vi "Actor Core.vi"(8 "error in":errorcluster, 11 "Nested in":refnum<class "Interactor.lvclass">) -> (0 "error out":errorcluster, 3 "Actor out":refnum<class "Actor.lvclass">)   [LabVIEW 2024, in "Interactor.lvlib" / "Interactor.lvclass"]
doc: "(<B>Filename</B>: Actor Framework.lvlib:Actor.lvclass:Actor Core.vi)\n\nReceives messages to the actor, reacts to them, and initiates any error handling that may shut the actor down.\n\nDescendant classes may override this VI to append parallel tasks for the actor to complete while it handles messages. Overrides use the Call Parent Method node."
uses:
  Interactor.lvclass
  <vilib>/ActorFramework/Actor/Actor.lvclass
  Object Dictionary UI/Object Dictionary UI.lvclass
  Home/Home.lvclass
  Interactor.lvclass/Interactor.ctl
  <vilib>/MGI/Panel Manager/Panel/Panel/Subpanel/Subpanel.lvclass
  <vilib>/ActorFramework/Stop Msg/Stop Msg.lvclass
  Interactor Messages/Show Nested Panel Msg/Show Nested Panel Msg.lvclass
  Interactor Messages/Publish Discovered Nodes Msg/Publish Discovered Nodes Msg.lvclass
  <vilib>/MGI/Panel Manager/Panel Actor/Panel Actor/Panel Actor.lvclass
  <vilib>/MGI/Panel Manager/Panel/Panel.lvlib
  CANopen Master/CANopen Master.lvclass
  HAL/Source/Instrument Manager/Instrument Manager.lvclass
  <vilib>/MGI/Panel Manager/Panel/Panel/Subpanel/Subpanel.vi
panel:
  in  "Copy Log Button":bool
  out "Communication Log":string
  in  "Object Dictionary":bool
  in  "Home Button":bool
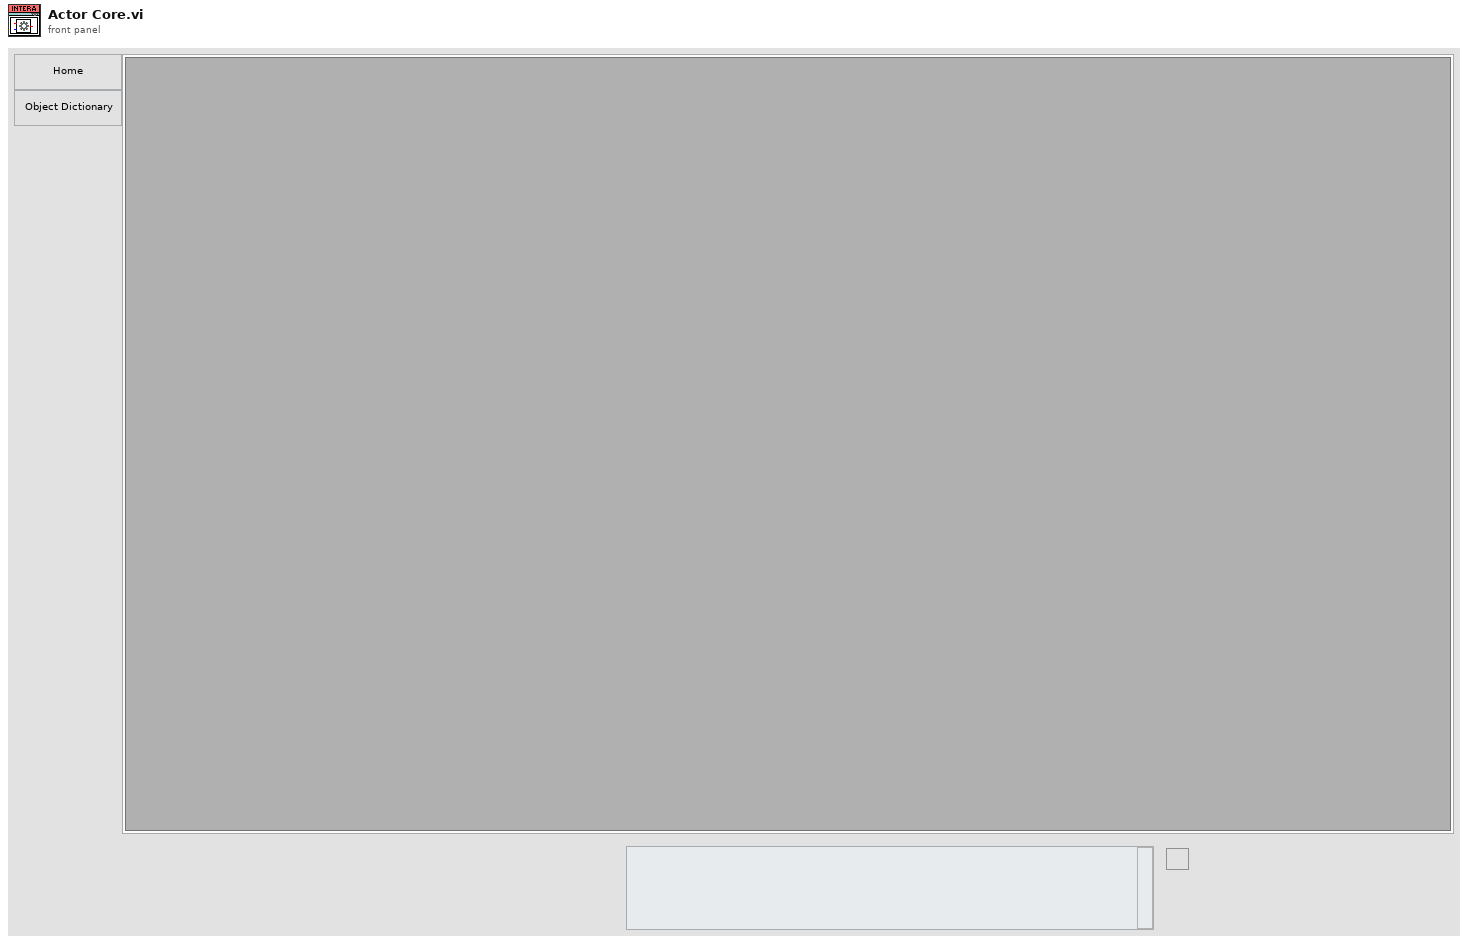
[diagram p1: front panel]
types:
  T1 = cluster{"Stop":refnum<user-event>, "Msg Sent Source":refnum<user-event>}
  T2 = cluster{"Stop CAN Task":refnum<user-event>, "Msg Received":refnum<user-event>, "CAN Task Error":refnum<user-event>, "Node Discovered":refnum<user-event>}
  T3 = cluster{"Pnl Actor":refnum<event-registration>, "Event Registration Refnum":refnum<event-registration>}
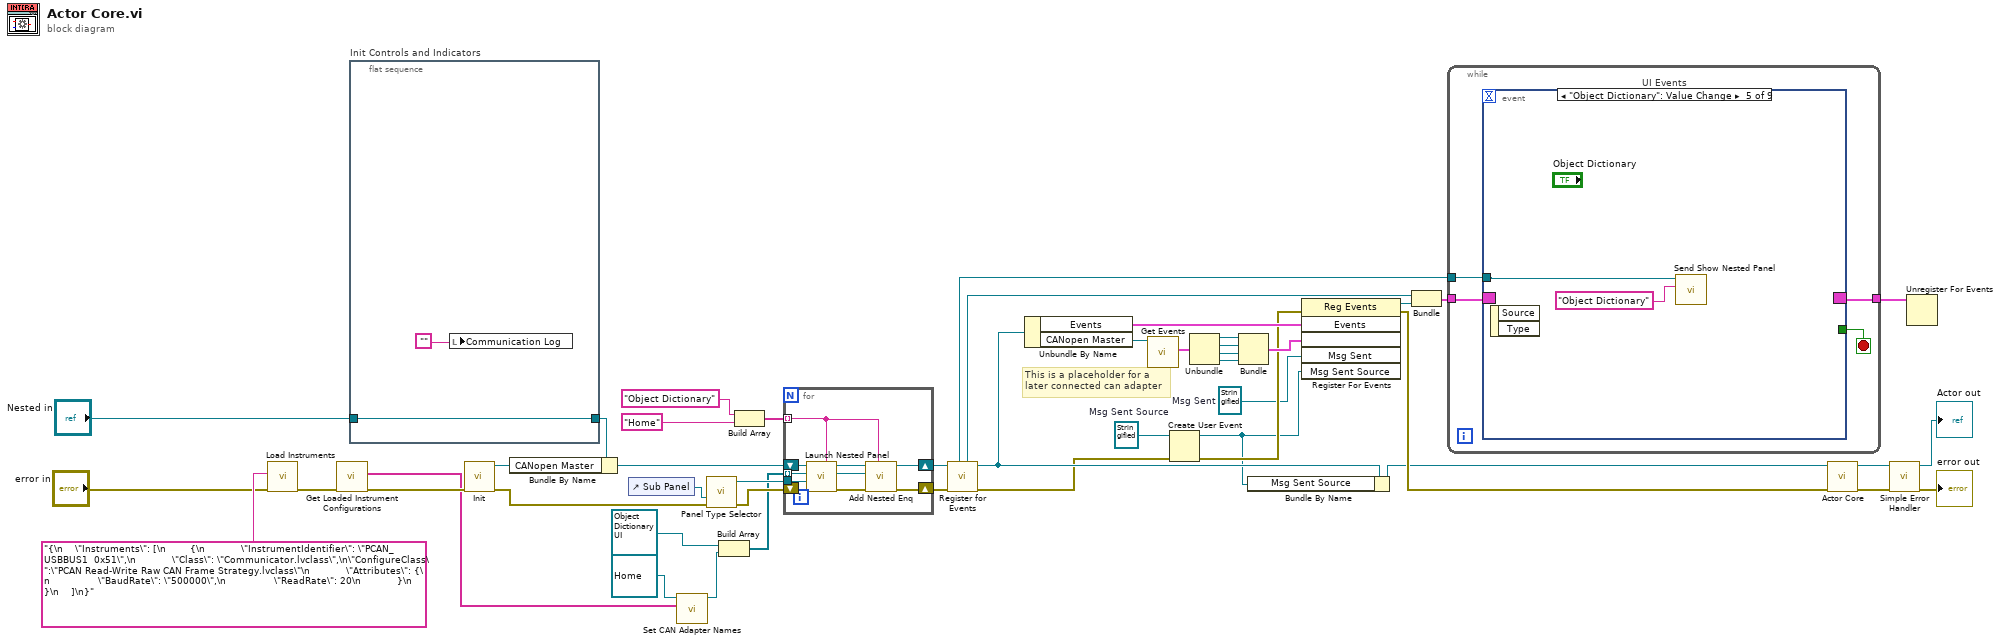
[diagram p0: block diagram]
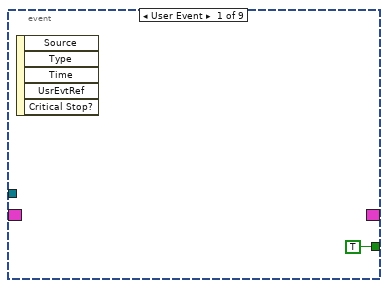
[diagram p2: hidden frame]
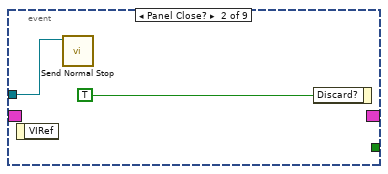
[diagram p3: hidden frame]
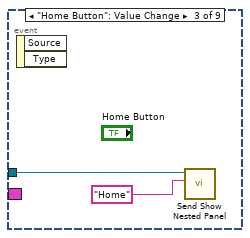
[diagram p4: hidden frame]
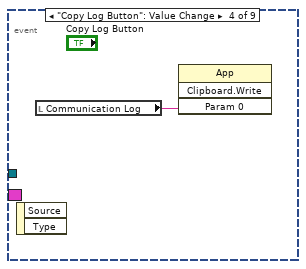
[diagram p5: hidden frame]
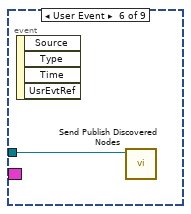
[diagram p6: hidden frame]
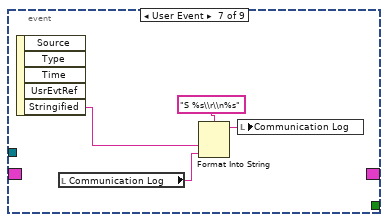
[diagram p7: hidden frame]
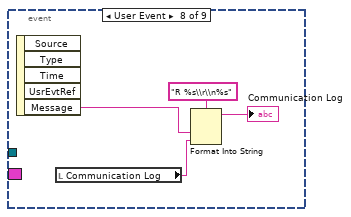
[diagram p8: hidden frame]
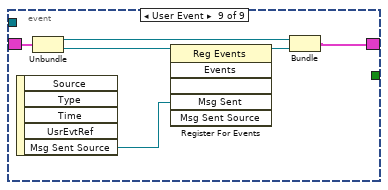
[diagram p9: hidden frame]
diagram:
  w5 = refnum<user-event> refnum  # Msg Sent Source
  w6 = refnum<user-event> refnum  # Msg Sent
  # "This is a placeholder for a\nlater connected can adapter"
  n1 = call "Load Instruments.vi"("Error In"="error in", "Source"="{\n    \"Instruments\": [\n        {\n            \"InstrumentIdentifier\": \"PCAN_USBBUS1  0x51\",\n            \"Class\": \"Communicator.lvclass\",\n\"ConfigureClass\":\"PCAN Read-Write Raw CAN Frame Strategy.lvclass\"\n            \"Attributes\": {\n                \"BaudRate\": \"500000\",\n                \"ReadRate\": 20\n            }\n        }\n    ]\n}" ("<JSON>CFG")) -> ("Error Out"=w13:errorcluster)  [unwired: 9 in]
  n2 = call "Get Loaded Instrument Configurations.vi"("Error In"=w13) -> ("Error Out"=w17:errorcluster, "Identifiers"=w16:string[])  [unwired: 8 in, 1 out]
  n3 = flat-sequence "Init Controls and Indicators" {
    tunnel: "Nested in" -> [w48]
    tunnel: [w48] -> w22
    frame #0 {
      n4 = local write "Communication Log"("") -> ()
    }
  }
  n5 = call "Init.vi"("error in"=w17) -> ("error out"=w19:errorcluster, "CANopen Master out"=w21:refnum<class "CANopen Master.lvclass">)  [unwired: 9 in]
  n6 = Bundle By Name(cluster=w22, "CANopen Master"=w21) -> (w20:refnum<class "Interactor.lvclass">)
  n7 = control-ref of="Sub Panel"() -> (w39:refnum<vi>)
  n8 = call "Set CAN Adapter Names.vi"("ICommunicate Names"=w16, "Home in"=refnum<class "Home.lvclass"> refnum) -> ("Home out"=w28:refnum<class "Home.lvclass">)  [unwired: 9 in]
  n9 = call-poly <vilib>:"Panel Type Selector.vi"("Error In"=w19, "Sub Panel"=w39) -> ("Error Out"=w38:errorcluster, "Subpanel Out"=w34:refnum<class "Subpanel.lvclass">)  [unwired: 8 in]
  n10 = Build Array(refnum<class "Object Dictionary UI.lvclass"> refnum ("Object Dictionary.lvlib:Object Dictionary.lvclass"), w28) -> (w33:refnum<class "Panel Actor.lvclass">[])
  n11 = Build Array("Object Dictionary" ("Debug Alias"), "Home" ("Debug Alias")) -> (w32:string[])
  n12 = for {
    tunnel: w34 -> [w51]
    shift-right: [w55] -> w37
    shift-left: w38 -> [w57]
    shift-right: [w52] -> w35
    shift-left: w20 -> [w56]
    tunnel: w33 -> [w50] mode=indexing
    tunnel: w32 -> [w49] mode=indexing
    n13 = call <vilib>:"Launch Nested Panel.vi"("Debug Alias"=w49, "error in (no error)"=w57, "Panel"=w51, "Nested Panel Actor"=w50, "Panel Actor in"=w56) -> ("error out"=w55:errorcluster, "Nested Actor's Enqueuer"=w53:refnum<class "Message Enqueuer.lvclass">, "Panel Actor out"=w54:refnum<class "Interactor.lvclass">)  [unwired: 3 in, 1 out]
    n14 = call "Add Nested Enq.vi"("Ident"=w49, "Nested Actor's Enqueuer"=w53, "Interactor in"=w54) -> ("Interactor out"=w52:refnum<class "Interactor.lvclass">)  [unwired: 8 in]
  }
  n15 = call <vilib>:"Register for Events.vi"("Error In"=w37, "Panel Actor in"=w35) -> ("Error Out"=w8:errorcluster, "Panel Actor out"=w36:refnum<class "Interactor.lvclass">, "Pnl Actor"=w40:refnum<event-registration>, "Self Enqueuer"=w43:refnum<class "Message Enqueuer.lvclass">)  [unwired: 6 in]
  n16 = Unbundle By Name(w36) -> ("Events"=w27:T1, "CANopen Master"=w23:refnum<class "CANopen Master.lvclass">)
  n17 = call "Get Events.vi"("CANopen Master in"=w23) -> ("Events"=w25:T2)  [unwired: 9 in, 1 out]
  n18 = Create User Event(user event datatype=w5, error in=w8) -> (user event=w3:refnum<user-event>, error out=w7:errorcluster)
  n19 = Unbundle(w25) -> ("Stop CAN Task"=w12:refnum<user-event>, "Msg Received"=w11:refnum<user-event>, "CAN Task Error"=w10:refnum<user-event>, "Node Discovered"=w9:refnum<user-event>)
  n20 = Bundle("Stop CAN Task"=w12, "Msg Received"=w11, "CAN Task Error"=w10, "Node Discovered"=w9) -> (w24:T2)  [unwired: 1 in]
  n21 = Bundle By Name(cluster=w36, "Msg Sent Source"=w3) -> (w4:refnum<class "Interactor.lvclass">)
  n22 = register-events ("Main Register for Events")(error in=w7, w27, w24, w6, w3) -> (reference out=w41:refnum<event-registration>, error out=w26:errorcluster)  [unwired: 1 in]
  n23 = Bundle("Pnl Actor"=w40, "Event Registration Refnum"=w41) -> (w42:T3)  [unwired: 1 in]
  n24 = while {
    tunnel: w42 -> [w61]
    tunnel: [w59] -> w44
    tunnel: w43 -> [w58]
    stop <- w60 stop-if-true
    n25 = event "UI Events" shown="[4] \"Object Dictionary\": Value Change" {
      selector: w61 -> [_ _ _ _ _ _ _ _ w84]
      dyn-events: [_ _ _ _ _ _ _ _ w79] -> w59
      timeout: _ -> [_ _ _ _ _ _ _ _ _]
      tunnel: [TRUE _ _ _ _ _ _ _ _] -> w60
      tunnel: w58 -> [_ w63 w66 _ w68 w70 _ _ _]
      event User Event {
        n26 = event-data() -> ()  [unwired: 1 in, 5 out]
      }
      event Panel Close? {
        n27 = event-data() -> ()  [unwired: 1 in, 1 out]
        n28 = call <vilib>:"Send Normal Stop.vi"("Message Enqueuer"=w63) -> ()  [unwired: 10 in, 1 out]
        n29 = event-data("Discard?"=TRUE) -> ()  [unwired: 1 in, 1 out]
      }
      event "Home Button": Value Change {
        n30 = event-data() -> ()  [unwired: 1 in, 2 out]
        n31 = call "Send Show Nested Panel.vi"("Ident"="Home", "Message Enqueuer"=w66) -> ()  [unwired: 8 in, 2 out]
      }
      event "Copy Log Button": Value Change {
        n32 = event-data() -> ()  [unwired: 1 in, 2 out]
        n33 = local read "Communication Log"() -> (w67:string)
        n34 = invoke class="App" method="Clipboard.Write"("Param 0"=w67) -> ()  [unwired: 3 in, 4 out]
      }
      event "Object Dictionary": Value Change {
        n35 = event-data() -> ()  [unwired: 1 in, 2 out]
        n36 = call "Send Show Nested Panel.vi"("Ident"="Object Dictionary", "Message Enqueuer"=w68) -> ()  [unwired: 8 in, 2 out]
      }
      event User Event {
        n37 = event-data() -> ()  [unwired: 1 in, 4 out]
        n38 = call "Send Publish Discovered Nodes.vi"("Message Enqueuer"=w70) -> ()  [unwired: 9 in, 2 out]
      }
      event User Event {
        n39 = event-data() -> ("Stringified"=w73:string)  [unwired: 1 in, 4 out]
        n40 = local read "Communication Log"() -> (w72:string)
        n41 = Format Into String(format string="S %s\\r\\n%s", w73, w72) -> (resulting string=w71:string)  [unwired: 2 in, 1 out]
        n42 = local write "Communication Log"(w71) -> ()
      }
      event User Event {
        n43 = event-data() -> ("Message"=w78:string)  [unwired: 1 in, 4 out]
        n44 = local read "Communication Log"() -> (w77:string)
        n45 = Format Into String(format string="R %s\\r\\n%s", w78, w77) -> (resulting string=→"Communication Log":string)  [unwired: 2 in, 1 out]
      }
      event User Event {
        n46 = event-data() -> ("Msg Sent Source"=w82:refnum<user-event>)  [unwired: 1 in, 4 out]
        n47 = Unbundle(w84) -> ("Pnl Actor"=w80:refnum<event-registration>, "Event Registration Refnum"=w83:refnum<event-registration>)
        n48 = register-events ("Main Register for Events")(reference=w83, w82) -> (reference out=w81:refnum<event-registration>)  [unwired: 4 in, 1 out]
        n49 = Bundle("Pnl Actor"=w80, "Event Registration Refnum"=w81) -> (w79:T3)  [unwired: 1 in]
      }
    }
  }
  n50 = call-parent "Actor Core.vi"("error in"=w26, "Panel Actor in"=w4) -> ("error out"=w46:errorcluster, "Actor out"=→"Actor out":refnum<class "Actor.lvclass">)  [unwired: 8 in]
  n51 = call <vilib>:"Simple Error Handler.vi"("error in (no error)"=w46) -> ("error out"=→"error out":errorcluster)  [unwired: 4 in, 4 out]
  n52 = Unregister For Events(event registration refnum=w44) -> ()  [unwired: 1 in, 1 out]
